vi "Do Turn.vi"(6 "Divisor":T1, 8 "error in (no error)":errorcluster, 11 "Monkey in":refnum<class "Monkey.lvclass">) -> (0 "error out":errorcluster, 1 "Item":T1, 2 "Dest":i32, 3 "Monkey out":refnum<class "Monkey.lvclass">, 4 "Throw?":bool, 5 "old":T1)   [LabVIEW 2022 SP3, in "AoC22.lvlib" / "Monkey.lvclass"]
uses:
  Monkey.lvclass
  Worry Level.ctl
  Monkey.lvclass/Monkey.ctl
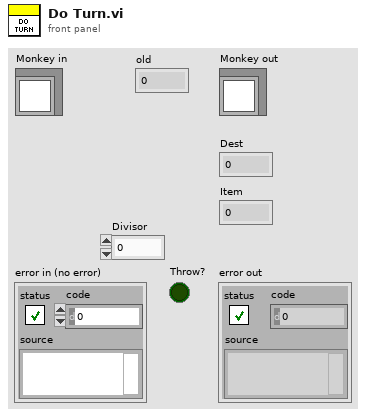
[diagram p1: front panel]
types:
  T1 = typedef "AoC22.lvlib/Monkey.lvclass/Worry Level.ctl" = u64
  T2 = typedef "AoC22.lvlib/Monkey.lvclass/Operation.ctl" = cluster{"Op":T3, "Val":T1}
  T3 = typedef "AoC22.lvlib/Monkey.lvclass/Op.ctl" = enum16{"+", "*"}
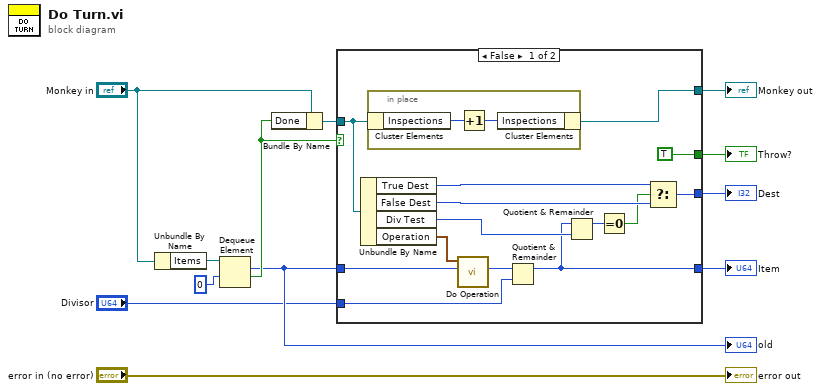
[diagram p0: block diagram]
diagram:
  n1 = Unbundle By Name("Monkey in") -> ("Items"=w11:refnum<queue>)
  n2 = Dequeue Element(queue=w11, timeout in ms (-1)=0) -> (element=w6:T1, timed out?=w7:bool)  [unwired: 1 in, 2 out]
  "old" <- w6
  n3 = Bundle By Name(cluster="Monkey in", "Done"=w7) -> (w8:refnum<class "Monkey.lvclass">)
  n4 = case shown="False" w7 {
    tunnel: w8 -> [w26 w29]
    tunnel: w6 -> [w17 _]
    tunnel: [w23 w29] -> w5
    tunnel: [w19 _] -> w4
    tunnel: [w13 _] -> w3
    tunnel: [TRUE _] -> w2
    tunnel: "Divisor" -> [w14 _]
    frame False {
      n5 = Unbundle By Name(w26) -> ("True Dest"=w25:i32, "False Dest"=w24:i32, "Div Test"=w22:T1, "Operation"=w18:T2)
      n6 = in-place {
        n7 = in-place-cluster #1(w26) -> ("Inspections"=w28:u64)
        n8 = Increment(x=w28) -> (x+1=w27:u64)
        n9 = in-place-cluster #1("Inspections"=w27) -> (w23:refnum<class "Monkey.lvclass">)
      }
      n10 = call "Do Operation.vi"("old"=w17, "Operation"=w18) -> ("new"=w15:T1)  [unwired: 9 in]
      n11 = Quotient & Remainder(x=w15, y=w14) -> (x-y*floor(x/y)=w13:T1)  [unwired: 1 out]
      n12 = Quotient & Remainder(x=w13, y=w22) -> (x-y*floor(x/y)=w21:T1)  [unwired: 1 out]
      n13 = Equal To 0?(x=w21) -> (x = 0?=w20:bool)
      n14 = Select(t=w25, s=w20, f=w24) -> (s? t:f=w19:i32)
    }
    frame True {
    }
  }
  "Monkey out" <- w5
  "Throw?" <- w2
  "Item" <- w3
  "Dest" <- w4
  "error out" <- "error in (no error)"
